vi "(SubVI)Scope_Stop.vi"(8 "error in (no error)":errorcluster caption="에러 입력(에러 없음)") -> (0 "error out":errorcluster caption="에러 출력")   [LabVIEW 2020]
uses:
  Serial/Controls/(Ctrl)Serial_FGV Function.ctl
  Serial/Controls/(Ctrl)Serial_Write Read Option.ctl
  Serial/Instance VIs/(SubVI)Serial_Write-Read.vi
panel:
  out "Read Data 2":u8[](array[numeric]) format="%02x"
  out "Read Data":u8[](array[numeric]) format="%02x"
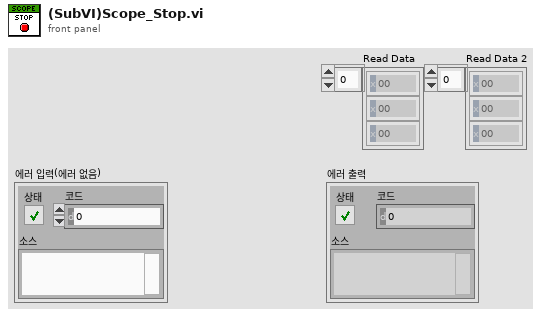
[diagram p1: front panel]
types:
  T1 = typedef "(Ctrl)Serial_Write Read Option.ctl" = cluster{"Echo Request":bool, "Header Verification":bool, "Checksum Verification":bool, "User Code Verifiaction":bool}
  T2 = typedef "(Ctrl)Serial_FGV Function.ctl" = enum16{"Initialize", "Read", "Read All", "Write", "Flush Buffer", "Get Ref.", "Close"}
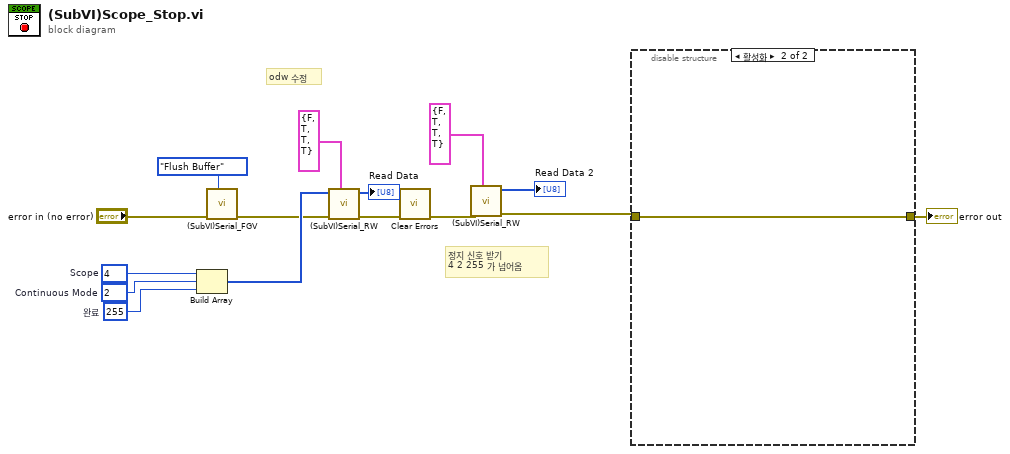
[diagram p0: block diagram]
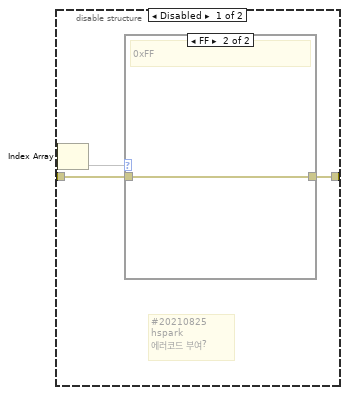
[diagram p2: hidden frame]
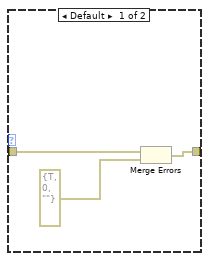
[diagram p3: hidden frame]
diagram:
  w14 = u8 2  # Continuous Mode
  w13 = u8 255  # 완료
  w15 = u8 4  # Scope
  # "정지 신호 받기\n4 2 255 가 넘어옴"
  # "odw 수정"
  n1 = Build Array(w15, w14, w13) -> (w10:u8[])
  n2 = call "(SubVI)Serial_FGV.vi"("Function"=(Ctrl)Serial_FGV_Function."Flush Buffer", "error in (no error)"="error in (no error)") -> ("error out"=w7:errorcluster)  [unwired: 7 in, 2 out]
  n3 = call-poly "(SubVI)Serial_RW.vi"("Option"=T1 {"Echo Request"=FALSE, "Header Verification"=TRUE, "Checksum Verification"=TRUE, "User Code Verifiaction"=TRUE}, "error in (no error)"=w7, "Data to Write"=w10) -> ("error out"=w5:errorcluster, "Read Data"=→"Read Data":u8[])  [unwired: 6 in, 1 out]
  n4 = call <vilib>:"Clear Errors.vi"("error in (no error)"=w5) -> ("error out"=w1:errorcluster)  [unwired: 5 in, 1 out]
  n5 = call-poly "(SubVI)Serial_RW.vi"("Option"=T1 {"Echo Request"=FALSE, "Header Verification"=TRUE, "Checksum Verification"=TRUE, "User Code Verifiaction"=TRUE}, "error in (no error)"=w1) -> ("error out"=w4:errorcluster, "Read Data"=→"Read Data 2":u8[])  [unwired: 7 in, 1 out]
  n6 = disable-structure shown="활성화" {
    disable-tunnel: [w18 w23] -> w11
    disable-tunnel: w4 -> [w17 w23]
    frame Disabled {
      # "#20210825\nhspark\n에러코드 부여?"
      n7 = Index Array() -> (element=w16)  [unwired: 2 in]
      n8 = case shown="FF" w16 {
        tunnel: w17 -> [w21 w22]
        tunnel: [w20 w22] -> w18
        frame Default {
          n9 = Merge Errors(w21, errorcluster {"status"=TRUE, "code"=0, "source"=""} ("에러 입력")) -> (w20:errorcluster)
        }
        frame 255 {
          # "0xFF"
        }
      }
    }
    frame Enabled {
    }
  }
  "error out" <- w11
